vi "Compuerta_BCheck.vi"(4 "BCHECK":bool, 6 "FALLA UU":bool, 8 "FALLA CD":bool, 9 "FALLA CU":bool, 10 "CONSOLIDACION":bool, 11 "SATURACION":bool) -> (3 "Boolean":bool)   [LabVIEW 2015]
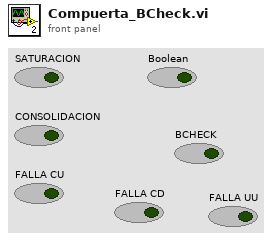
[diagram p1: front panel]
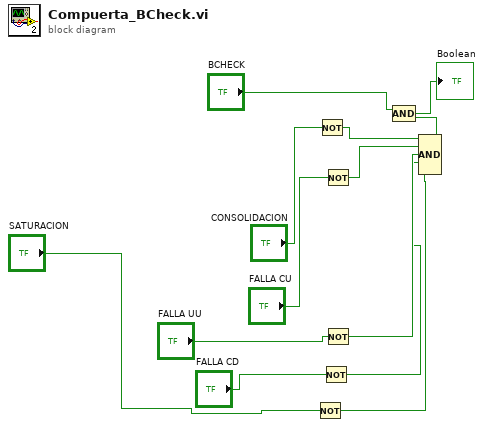
[diagram p0: block diagram]
diagram:
  n1 = Not(x="SATURACION") -> (.not. x?=w5:bool)
  n2 = Not(x="CONSOLIDACION") -> (.not. x?=w9:bool)
  n3 = Not(x="FALLA CD") -> (.not. x?=w6:bool)
  n4 = Not(x="FALLA CU") -> (.not. x?=w8:bool)
  n5 = Not(x="FALLA UU") -> (.not. x?=w7:bool)
  n6 = Compound Arithmetic op=AND(w9, w8, w7, w6, w5) -> (w10:bool)
  n7 = Compound Arithmetic op=AND("BCHECK", w10) -> (→"Boolean":bool)
